vi "Initialise Aircraft.vi"(8 "error IO":errorcluster, 11 "Aircraft ID":u8) -> (0 "error out":errorcluster)   [LabVIEW 2014]
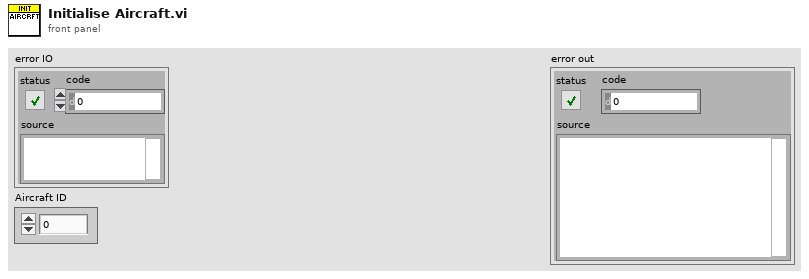
[diagram p1: front panel]
types:
  T1 = enum16{"ALL", "RAW_SENSORS", "EXTENDED_STATUS", "RC_CHANNELS", "RAW_CONTROLLER", "POSITION", "EXTRA1", "EXTRA2", "EXTRA3"}
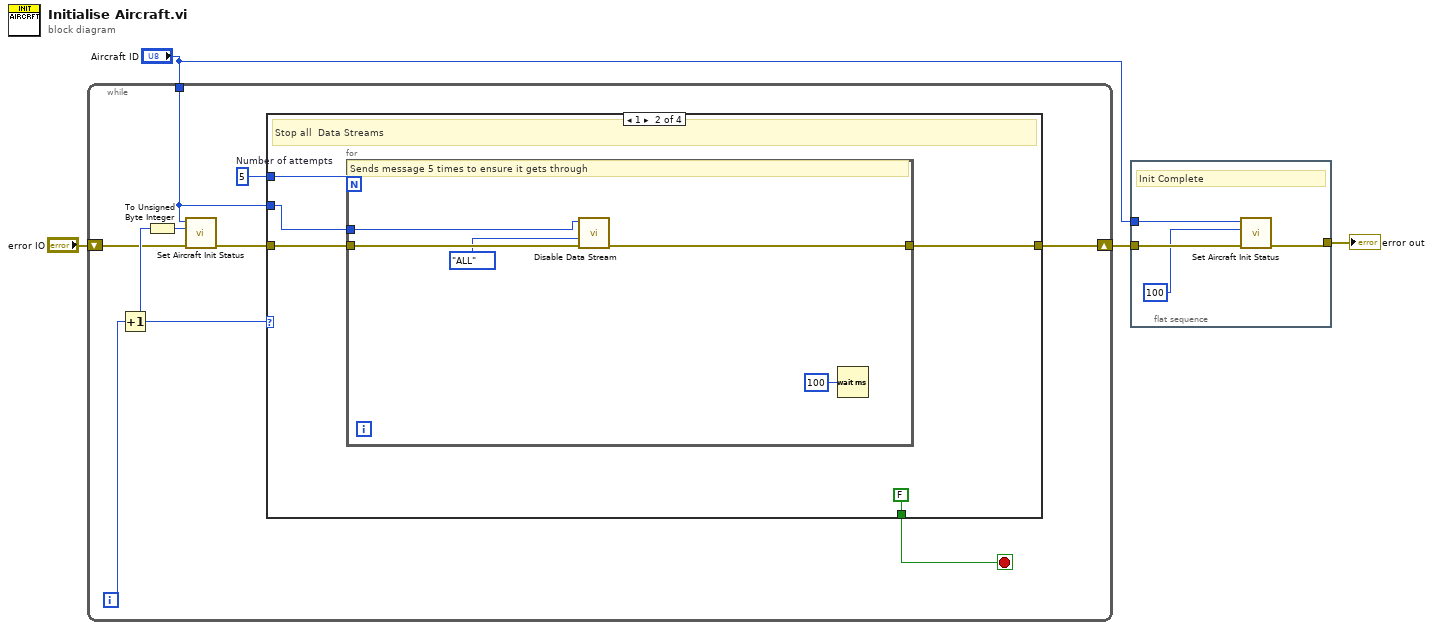
[diagram p0: block diagram]
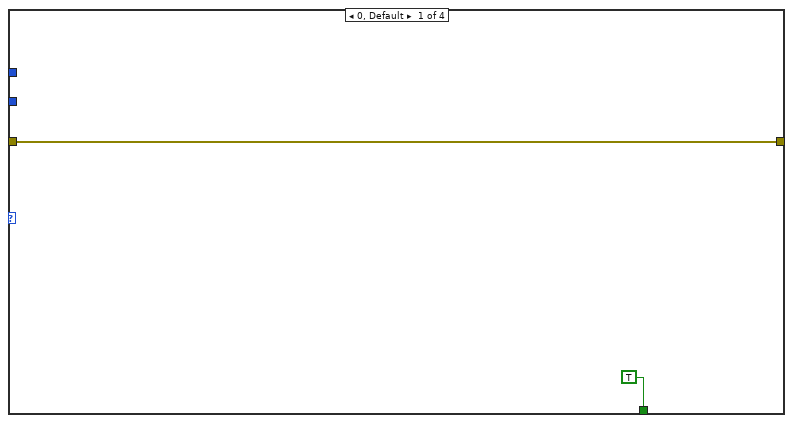
[diagram p2: hidden frame]
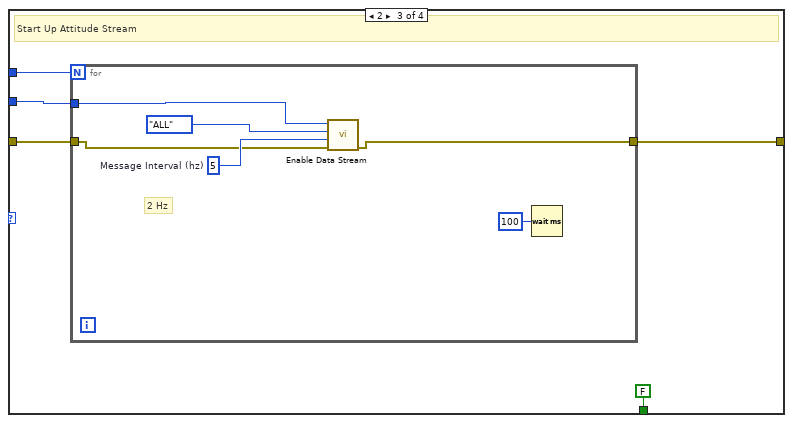
[diagram p3: hidden frame]
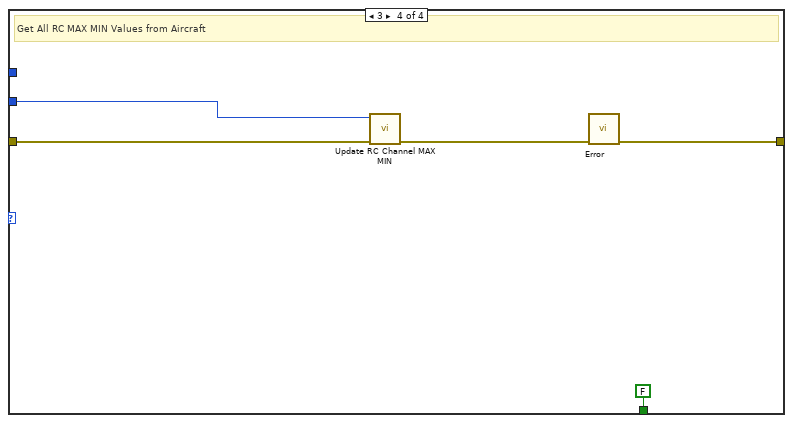
[diagram p4: hidden frame]
diagram:
  n1 = while {
    shift-right: [w5] -> w4
    shift-left: "error IO" -> [w9]
    tunnel: "Aircraft ID" -> [w7]
    i -> [w12]
    stop <- w13 stop-if-true
    w6 = 5  # Number of attempts
    n2 = Increment(x=w12) -> (x+1=w11:i32)
    n3 = To Unsigned Byte Integer(number=w11) -> (unsigned 8bit integer=w8:u8)
    n4 = call "Set Aircraft Init Status.vi"("Error In"=w9, "Initialisation"=w8, "Aircraft ID"=w7) -> ("Error Out"=w10:errorcluster)  [unwired: 8 in]
    n5 = case shown="1" w11 {
      tunnel: [TRUE FALSE FALSE FALSE] -> w13
      tunnel: [w14 w16 w26 w37] -> w5
      tunnel: w10 -> [w14 w19 w30 w40]
      tunnel: w7 -> [_ w18 w28 w38]
      tunnel: w6 -> [_ w17 w27 _]
      frame 0, Default {
      }
      frame 1 {
        # "Stop all  Data Streams"
        n6 = for {
          N: w17 -> [_]
          tunnel: w19 -> [w24]
          tunnel: w18 -> [w23]
          tunnel: [w22] -> w16
          # "Sends message 5 times to ensure it gets through"
          n7 = call "Disable Data Stream.vi"("error in (no error)"=w24, "req_stream_id"=T1."ALL", "Aircraft ID"=w23) -> ("error out"=w22:errorcluster)  [unwired: 8 in]
          n8 = Wait (ms)(milliseconds to wait=u32 100) -> ()  [unwired: 1 out]
        }
      }
      frame 2 {
        # "Start Up Attitude Stream"
        n9 = for {
          N: w27 -> [_]
          tunnel: w30 -> [w32]
          tunnel: w28 -> [w35]
          tunnel: [w31] -> w26
          w33 = u16 5  # Message Interval (hz)
          # "2 Hz"
          n10 = call "Enable Data Stream.vi"("error in (no error)"=w32, "Message Interval (hz)"=w33, "req_stream_id"=T1."ALL", "Aircraft Index"=w35) -> ("error out"=w31:errorcluster)  [unwired: 7 in]
          n11 = Wait (ms)(milliseconds to wait=u32 100) -> ()  [unwired: 1 out]
        }
      }
      frame 3 {
        # "Get All RC MAX MIN Values from Aircraft"
        n12 = call "Update RC Channel MAX MIN.vi"("Error In"=w40, "Aircraft ID"=w38) -> ("error out"=w39:errorcluster)  [unwired: 9 in]
        n13 = call "Error.vi"("Error In"=w39) -> ("Error Out"=w37:errorcluster)  [unwired: 10 in]
      }
    }
  }
  n14 = flat-sequence {
    tunnel: w4 -> [w45]
    tunnel: [w44] -> w3
    tunnel: "Aircraft ID" -> [w42]
    frame #0 {
      # "Init Complete"
      n15 = call "Set Aircraft Init Status.vi"("Error In"=w45, "Initialisation"=u8 100 ("Initalize"), "Aircraft ID"=w42) -> ("Error Out"=w44:errorcluster)  [unwired: 8 in]
    }
  }
  "error out" <- w3
